vi "Init Viewport.vi"(5 "Label":string, 8 "error in (no error)":errorcluster, 10 "Items":refnum<class "IObject.lvclass">[](array[class])) -> (0 "error out":errorcluster, 3 "Viewport out":refnum<class "Viewport.lvclass">)   [LabVIEW 2013, in "Viewport.lvclass"]
doc: "Copyright 2018, Wiebe Walstra, wiebe@carya.nl."
uses:
  Viewport.lvclass
  IObject.lvclass
  IContainer.lvclass
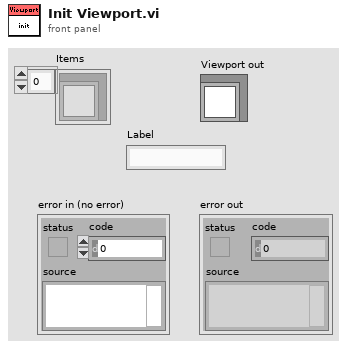
[diagram p1: front panel]
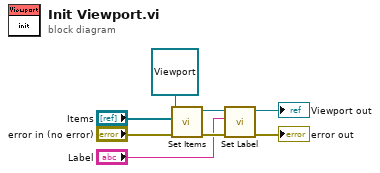
[diagram p0: block diagram]
diagram:
  n1 = call "Set Items.vi"("error in (no error)"="error in (no error)", "Items"="Items", "IContainer in"=refnum<class "Viewport.lvclass"> refnum ("Viewport in")) -> ("error out"=w7:errorcluster, "IContainer out"=w4:refnum<class "Viewport.lvclass">)  [unwired: 7 in]
  n2 = call "Set Label.vi"("error in (no error)"=w7, "Label"="Label", "MMI Scaling in"=w4) -> ("error out"=→"error out":errorcluster, "MMI Scaling out"=→"Viewport out":refnum<class "Viewport.lvclass">)  [unwired: 7 in]
